vi "Initialize Adpater Module.vi"(7 "Timeout (s)":dbl=5.0 caption="Time Target (s)", 8 "error in":errorcluster, 11 "FPGA VI Reference In":refnum<k20>) -> (0 "error out":errorcluster, 2 "FAM Configured":bool=TRUE, 3 "FPGA VI Reference Out":refnum<k20>)   [LabVIEW 2012, in "FlexRIO Host Library (User).lvlib"]
doc: "This VI initializes adpater mddule"
uses:
  <userlib>/FlexRIO Host Library/FlexRIO Host Library (User).lvlib
  <vilib>/rvi/errors/niLvFpgaAdjustHostInterfaceError.vi
  <vilib>/LabVIEW Targets/FPGA/FlexRIO/CustomFPGAMethods/79XXR_Method_IOModuleStatusImpl.vi
  <vilib>/rvi/interface/nirviReadWriteControl/nirviReadWriteControl.xnode
  <vilib>/rvi/interface/nirviMethod/nirviMethod.xnode
  NiFpgaLv.dll
  <vilib>/rvi/interface/Simulation/niFpgaSimulationCallBeginRW.vi
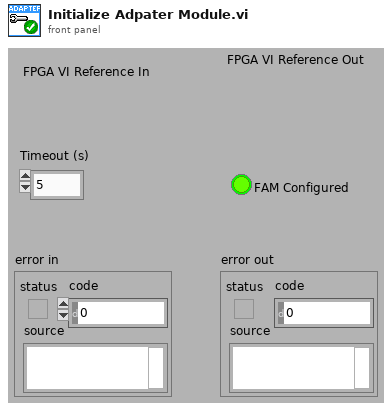
[diagram p1: front panel]
types:
  T1 = cluster{"io mod.initialization done":bool, "io mod.configuration error":bool, "io mod.synthesizer locked":bool, "io mod.spi idle":bool}
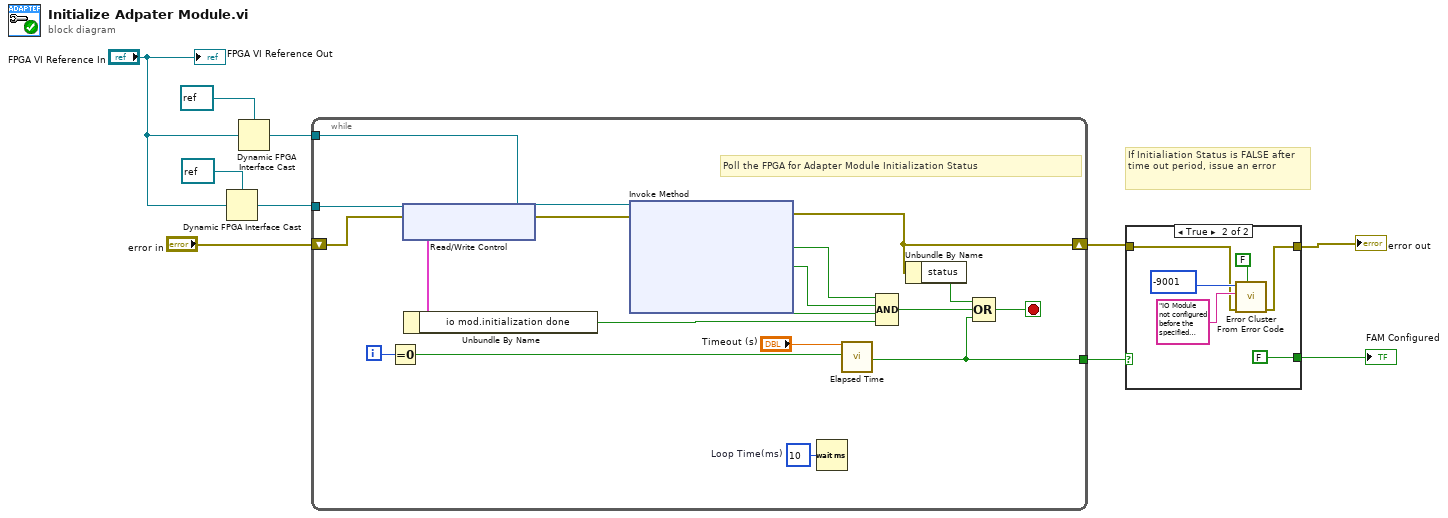
[diagram p0: block diagram]
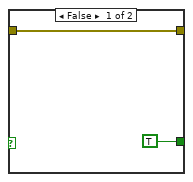
[diagram p2: hidden frame]
diagram:
  # "If Initialiation Status is FALSE after time out period, issue an error"
  n1 = Dynamic FPGA Interface Cast(Session In=refnum<k20> refnum ("Type"), Type="FPGA VI Reference In") -> (Session Out=w5:refnum<k20>)
  n2 = Dynamic FPGA Interface Cast(Session In=refnum<k20> refnum ("Type"), Type="FPGA VI Reference In") -> (Session Out=w1:refnum<k20>)
  n3 = while {
    shift-right: [w23] -> w9
    shift-left: "error in" -> [w16]
    tunnel: [w24] -> w8
    tunnel: w5 -> [w17]
    tunnel: w1 -> [w13]
    i -> [w12]
    stop <- w27 stop-if-true
    w28 = u32 10  # Loop Time(ms)
    # "Poll the FPGA for Adapter Module Initialization Status"
    n4 = Equal To 0?(x=w12) -> (x = 0?=w11:bool)
    n5 = xnode "Read/Write Control"("FPGA VI Reference In"=w17, "error in"=w16) -> ("error out"=w15:errorcluster, "IO Module Status"=w14:T1)  [unwired: 1 out]
    n6 = Unbundle By Name(w14) -> ("io mod.initialization done"=w18:bool)
    n7 = xnode "Invoke Method"("FPGA VI Reference In"=w13, "error in"=w15) -> ("error out"=w23:errorcluster, "IO Module Present?"=w21:bool, "Power Enabled?"=w20:bool, "IO Enabled?"=w19:bool)  [unwired: 2 out]
    n8 = Wait (ms)(milliseconds to wait=w28) -> ()  [unwired: 1 out]
    n9 = call "Elapsed Time"("Time Target (s)"="Timeout (s)", "Reset"=w11) -> ("Time has Elapsed"=w24:bool)  [unwired: 10 in, 7 out]
    n10 = Compound Arithmetic op=AND(w21, w20, w19, w18) -> (w22:bool)
    n11 = Unbundle By Name(w23) -> ("status"=w26:bool)
    n12 = Compound Arithmetic op=OR(w26, w22, w24) -> (w27:bool)
  }
  n13 = case shown="True" w8 {
    tunnel: w9 -> [w30 w32]
    tunnel: [w30 w35] -> w7
    tunnel: [TRUE ("Master FAM Configured") FALSE ("Master FAM Configured")] -> w6
    frame False {
    }
    frame True {
      n14 = call <vilib>:"Error Cluster From Error Code.vi"("show call chain? (False)"=FALSE, "error in (no error)"=w32, "error message (\"\")"="IO Module not configured before the specified timeout." ("source"), "error code (0)"=-9001 ("code")) -> ("error out"=w35:errorcluster)  [unwired: 5 in]
    }
  }
  "error out" <- w7
  "FAM Configured" <- w6
  "FPGA VI Reference Out" <- "FPGA VI Reference In"
